vi "Panel.vi"() -> ()   [LabVIEW 2021]
uses:
  Mete.ctl
  R.ctl
  P.ctl
  N.ctl
  D.ctl
  Odo Velocity.ctl
panel:
  out "Km/h":T1 scale=0.0..200.0
  in  "stop":bool
  in  "Slide":u32(slide) max=900 scale=0.0..999.0
  in  "Boolean 8":bool
  in  "Boolean 7":bool
  in  "Boolean 6":bool
  in  "Boolean 5":bool
  out "Boolean 4":T2
  out "Boolean 3":T3
  out "Boolean 2":T4
  out "Boolean":T5
  out "Gauge":T6 scale=0.0..900.0
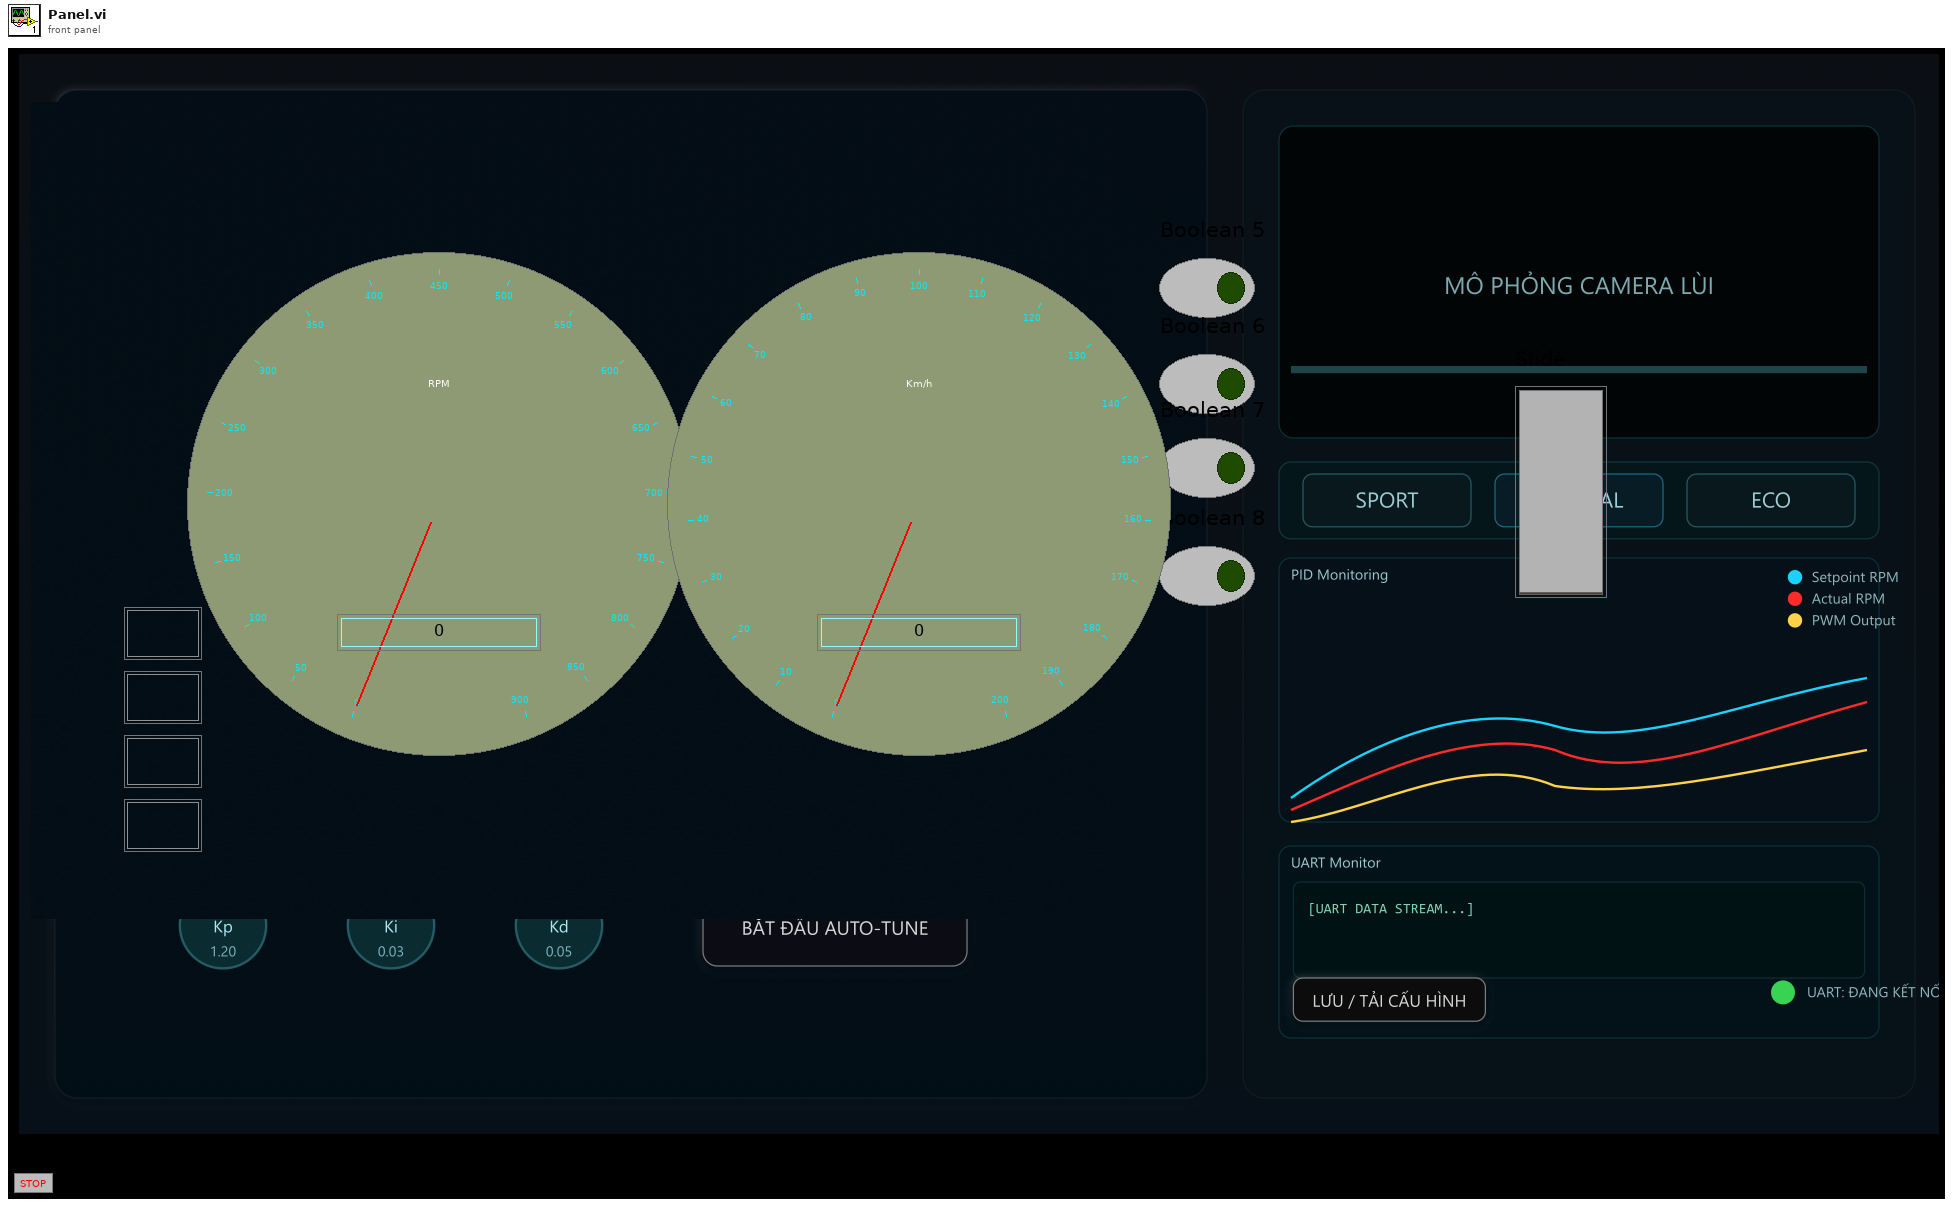
[diagram p1: front panel]
types:
  T1 = typedef "Odo Velocity.ctl" = u16
  T2 = typedef "D.ctl" = bool
  T3 = typedef "N.ctl" = bool
  T4 = typedef "P.ctl" = bool
  T5 = typedef "R.ctl" = bool
  T6 = typedef "Mete.ctl" = u16
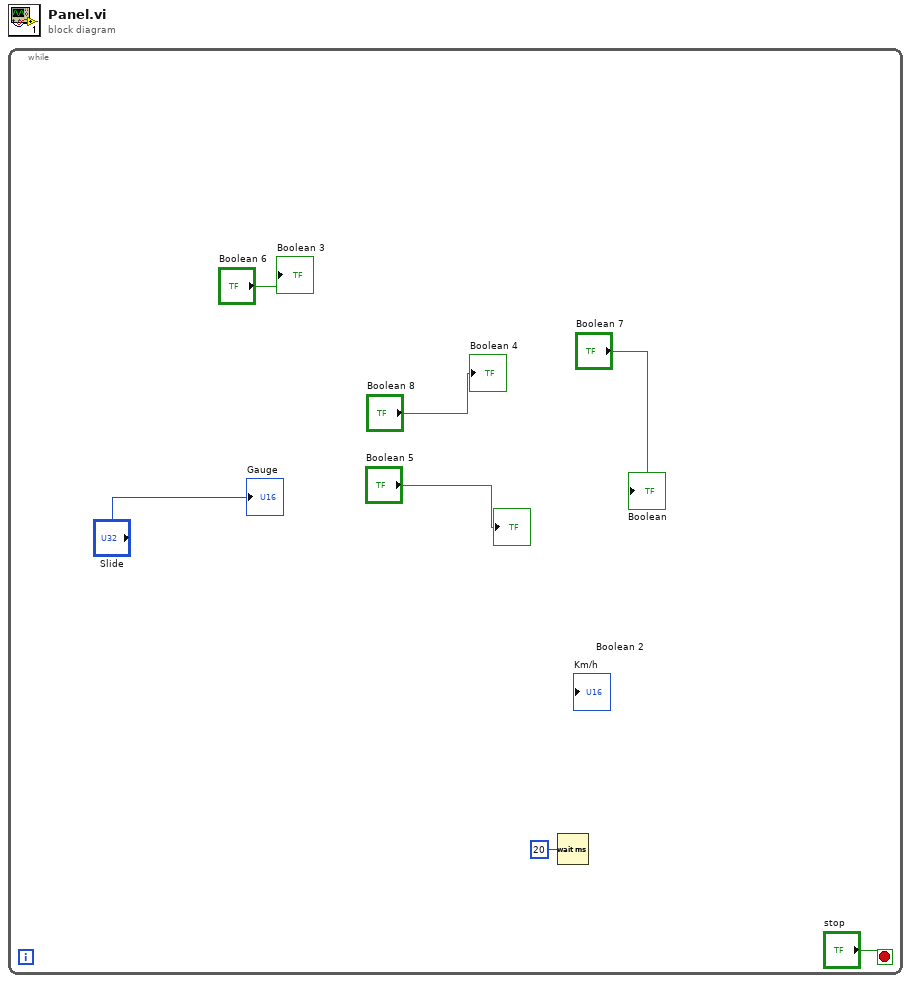
[diagram p0: block diagram]
diagram:
  n1 = while {
    stop <- "stop" stop-if-true
    n2 = Wait (ms)(milliseconds to wait=u32 20) -> ()  [unwired: 1 out]
    "Gauge" <- "Slide"
    "Boolean 2" <- "Boolean 5"
    "Boolean 3" <- "Boolean 6"
    "Boolean" <- "Boolean 7"
    "Boolean 4" <- "Boolean 8"
  }
